vi "gui_checkEmergencyStop.vi"(7 "Check":bool, 8 "error in (no error)":errorcluster, 11 "modbusData":refnum<notifier>) -> (0 "error out":errorcluster, 4 "Stop":bool, 5 "Continue check":bool)   [LabVIEW 2019]
uses:
  instrument/instr_dataCluster.ctl
  instrument/Instrument.lvclass
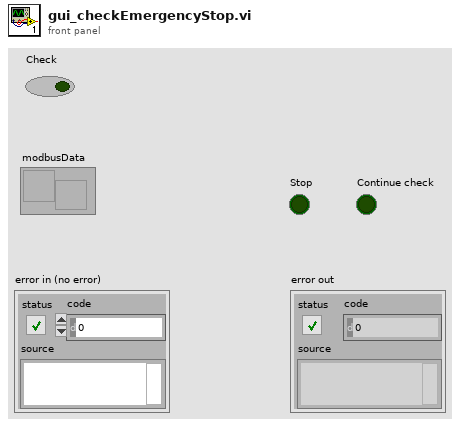
[diagram p1: front panel]
types:
  T1 = typedef "Instrument.lvclass/instr_dataCluster.ctl" = cluster{"电源电压 V":dbl, "电源电流A":dbl, "扭矩N/m":dbl, "速度r/M":dbl, "温度℃":dbl[], "流量计L/M":dbl[]}
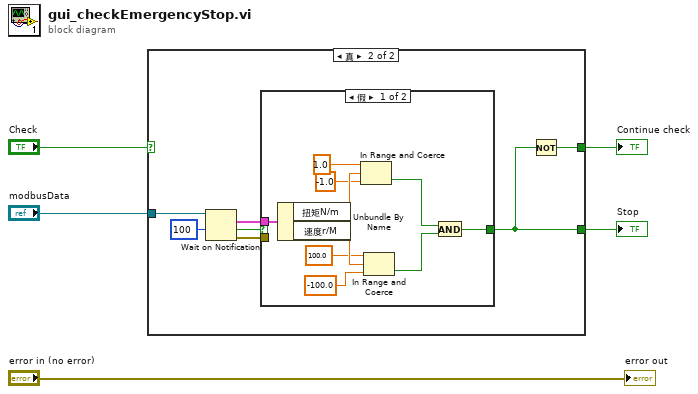
[diagram p0: block diagram]
diagram:
  n1 = case shown="真" "Check" {
    selector: "Check" -> [w6 _]
    tunnel: "modbusData" -> [_ w13]
    tunnel: [w6 w8] -> w3
    tunnel: [w6 w7] -> w2
    frame False {
    }
    frame True {
      n2 = Wait on Notification(notifier=w13, timeout in ms (-1)=100) -> (notification=w9:T1, timed out?=w11:bool, error out=w10:errorcluster)  [unwired: 2 in, 1 out]
      n3 = case shown="假" w11 {
        selector: w11 -> [_ w24]
        tunnel: w10 -> [_ _]
        tunnel: [w16 w24] -> w7
        tunnel: w9 -> [w23 _]
        frame False {
          n4 = Unbundle By Name(w23) -> ("扭矩N/m"=w22:dbl, "速度r/M"=w21:dbl)
          n5 = In Range and Coerce(upper limit=1.0, x=w22, lower limit=-1.0) -> (In Range?=w15:bool)  [unwired: 1 out]
          n6 = In Range and Coerce(upper limit=100.0, x=w21, lower limit=-100.0) -> (In Range?=w14:bool)  [unwired: 1 out]
          n7 = And(x=w15, y=w14) -> (x .and. y?=w16:bool)
        }
        frame True {
        }
      }
      n8 = Not(x=w7) -> (.not. x?=w8:bool)
    }
  }
  "Stop" <- w2
  "Continue check" <- w3
  "error out" <- "error in (no error)"
